vi "Read Current.vi"(8 "error in (no error)":errorcluster, 11 "Simple Device in":refnum<class "Simple Device.lvclass">) -> (0 "error out":errorcluster, 2 "Current [mA]":dbl, 3 "Simple Device out":refnum<class "Simple Device.lvclass">)   [LabVIEW 2020, in "Simple Device.lvclass"]
uses:
  Simple Device.lvclass
  Simple Device.lvclass/Simple Device.ctl
  TALOS/TALOS_PPL.lvlibp
  DeviceSim.lvlibp/DeviceReference/Simple  Virtual Device.lvclass
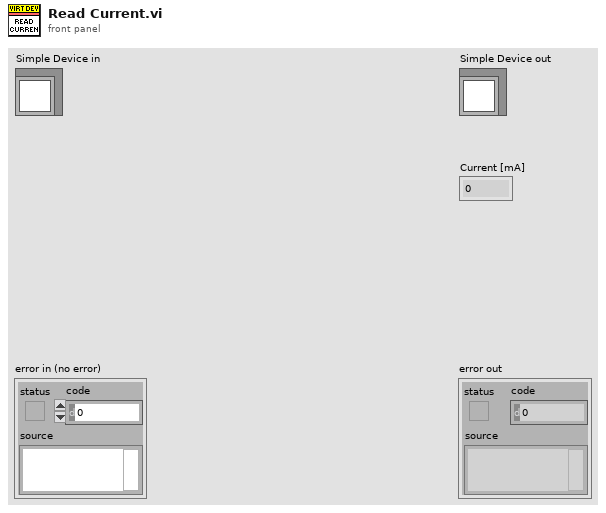
[diagram p1: front panel]
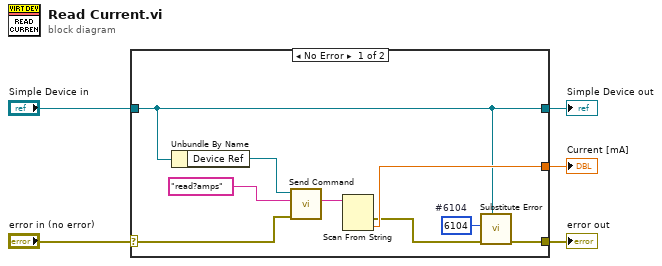
[diagram p0: block diagram]
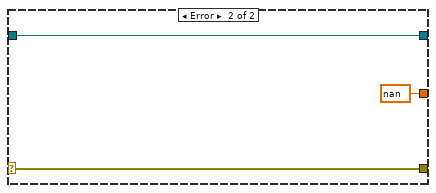
[diagram p2: hidden frame]
diagram:
  n1 = case shown="No Error" "error in (no error)" {
    selector: "error in (no error)" -> [w7 w17]
    tunnel: [w12 w17] -> w4
    tunnel: [w11 w16] -> w2
    tunnel: "Simple Device in" -> [w11 w16]
    tunnel: [w14 nan] -> w1
    frame No Error {
      w10 = 6104  # #6104
      n2 = Unbundle By Name(w11) -> ("Device Ref"=w9:refnum<data-value>)
      n3 = call "Send Command.vi"("error in (no error)"=w7, "Command"="read?amps", "Device Ref in"=w9) -> ("Response"=w6:string)  [unwired: 6 in, 2 out]
      n4 = Scan From String(input string=w6) -> (error out=w13:errorcluster, output 1=w14:dbl)  [unwired: 4 in, 2 out]
      n5 = call "Substitute Error.vi"("LabVIEW Object"=w11, "error in (no error)"=w13, "Error Code"=w10) -> ("error out"=w12:errorcluster)  [unwired: 8 in]
    }
    frame Error {
    }
  }
  "error out" <- w4
  "Simple Device out" <- w2
  "Current [mA]" <- w1
